vi "NiFPGA Wait On IRQs.vi"(6 "Timeout":u32, 8 "error in (no error)":errorcluster, 9 "IRQs":u32, 10 "Context":u32, 11 "Session In":u32) -> (0 "error out":errorcluster, 1 "IRQs Asserted":u32, 3 "Session Out":u32, 4 "Timed Out?":bool)   [LabVIEW 2010, in "FPGA Interface Wrapper.lvlib"]
doc: "This is a blocking function that stops the calling thread until the FPGA asserts any IRQ in the irqs parameter, or until the function call times out. Before calling this function, you must use NiFpga_ReserveIrqContext to reserve an IRQ context. No other threads can use the same context when this function is called. You can use the irqsAsserted parameter to determine which IRQs were asserted for each function call."
uses:
  <userlib>/_FPGA Interface Advanced Tools/FPGA Interface Wrapper/FPGA Interface Wrapper.lvlib
  NiFpga.dll
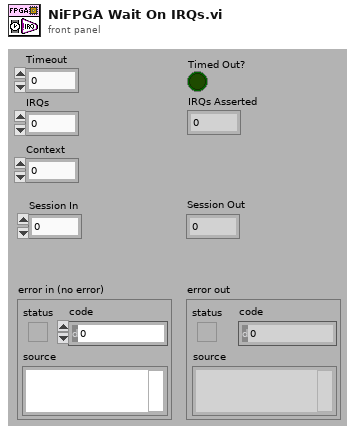
[diagram p1: front panel]
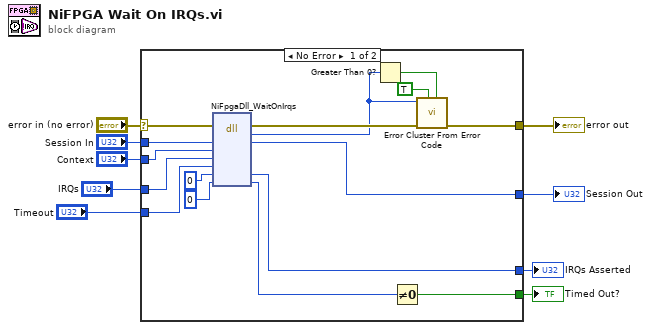
[diagram p0: block diagram]
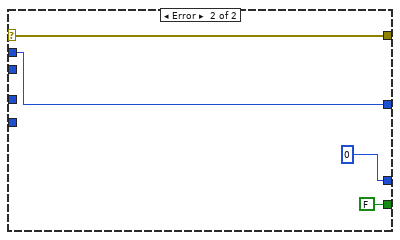
[diagram p2: hidden frame]
diagram:
  n1 = case shown="No Error" "error in (no error)" {
    selector: "error in (no error)" -> [w25 w28]
    tunnel: [w10 w28] -> w9
    tunnel: [w24 w29] -> w7
    tunnel: "Session In" -> [w23 w29]
    tunnel: "Context" -> [w18 _]
    tunnel: [w21 FALSE] -> w4
    tunnel: [w20 u32 0 ("Context")] -> w3
    tunnel: "Timeout" -> [w19 _]
    tunnel: "IRQs" -> [w17 _]
    frame No Error {
      n2 = dll-call lib="NiFpga.dll" fn="NiFpgaDll_WaitOnIrqs"(error in=w25, "Session"=w23, "Context"=w18, "IRQs"=w17, "Timeout"=w19, "IRQs Asserted"=u32 0, "Timed Out?"=u8 0) -> (error out=w12:errorcluster, "Status"=w11:i32, "Session"=w24:u32, "IRQs Asserted"=w20:u32, "Timed Out?"=w22:u8)  [unwired: 5 in, 1 out]
      n3 = Greater Than 0?(x=w11) -> (x > 0?=w13:bool)
      n4 = Not Equal To 0?(x=w22) -> (x != 0?=w21:bool)
      n5 = call <vilib>:"Error Cluster From Error Code.vi"("is warning? (False)"=w13, "show call chain? (False)"=TRUE, "error in (no error)"=w12, "error code (0)"=w11) -> ("error out"=w10:errorcluster)  [unwired: 5 in]
    }
    frame Error {
    }
  }
  "error out" <- w9
  "Session Out" <- w7
  "Timed Out?" <- w4
  "IRQs Asserted" <- w3
